vi "Camera Global.vi"() -> ()   [LabVIEW 2013]
panel:
  in  "Front Camera":T1
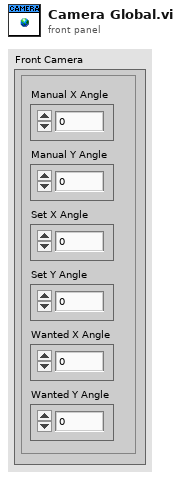
[diagram p1: front panel]
types:
  T1 = cluster{"Manual X Angle":dbl, "Manual Y Angle ":dbl, "Set X Angle":dbl, "Set Y Angle ":dbl, "Wanted X Angle":dbl, "Wanted Y Angle  ":dbl}
diagram:
